vi "get_output_type.vi"(8 "error in (no error)":errorcluster, 11 "DAQmxWriteSignals.lvclass in":refnum<class "SignalWriterDL090202DAQmx.lvclass">) -> (0 "error out":errorcluster, 2 "output type":T1, 3 "DAQmxWriteSignals.lvclass out":refnum<class "SignalWriterDL090202DAQmx.lvclass">)   [LabVIEW 2010, in "SignalWriterDL090202DAQmx.lvclass"]
uses:
  SignalWriterDL090202DAQmx.lvclass
  output_type_enum.ctl
  SignalWriterDL090202DAQmx.lvclass/SignalWriterDL090202DAQmx.ctl
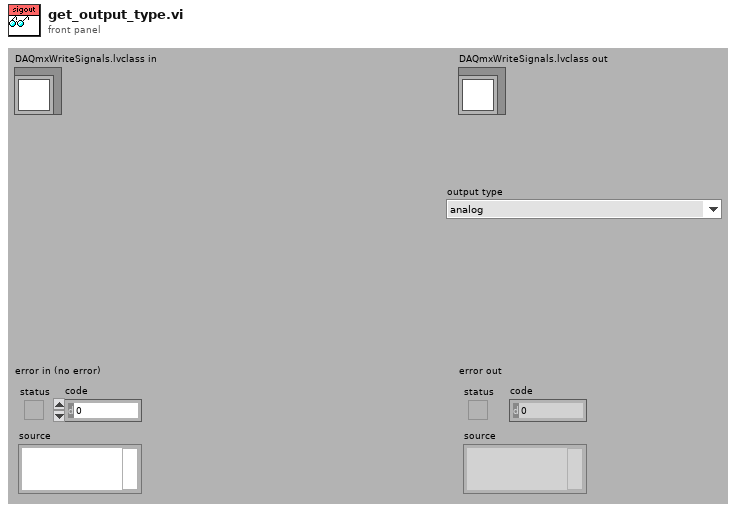
[diagram p1: front panel]
types:
  T1 = typedef "SignalWriterDL090202DAQmx.lvclass/output_type_enum.ctl" = enum16{"analog", "digital (U8)", "digital (U16)", "digital (U32)"}
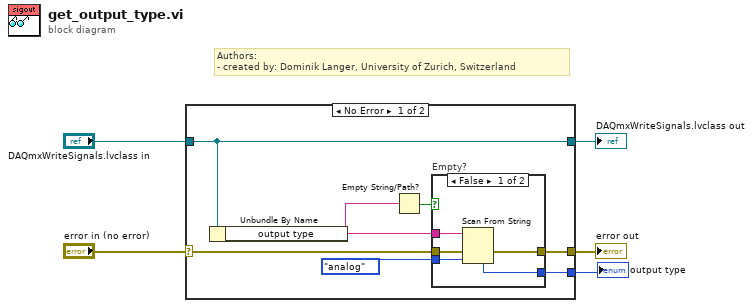
[diagram p0: block diagram]
diagram:
  # "Authors: \n- created by: Dominik Langer, University of Zurich, Switzerland"
  n1 = case shown="No Error" "error in (no error)" {
    selector: "error in (no error)" -> [w11 w20]
    tunnel: [w10 w20] -> w4
    tunnel: [w12 w21] -> w2
    tunnel: "DAQmxWriteSignals.lvclass in" -> [w12 w21]
    tunnel: [w8 _] -> w1
    frame No Error {
      n2 = Unbundle By Name(w12) -> ("output type"=w7:string)
      n3 = Empty String/Path?(string/path=w7) -> (empty?=w6:bool)
      n4 = case "Empty?" shown="False" w6 {
        tunnel: w11 -> [w17 w19]
        tunnel: [w16 w19] -> w10
        tunnel: output_type_enum."analog" ("output type") -> [w15 w18]
        tunnel: [w14 w18] -> w8
        tunnel: w7 -> [w13 _]
        frame False {
          n5 = Scan From String(input string=w13, error in=w17, default 1=w15) -> (error out=w16:errorcluster, output 1=w14:T1)  [unwired: 2 in, 2 out]
        }
        frame True {
        }
      }
    }
    frame Error {
    }
  }
  "error out" <- w4
  "DAQmxWriteSignals.lvclass out" <- w2
  "output type" <- w1
